vi "Configure Channels.vi"(8 "error in":errorcluster, 11 "AI DAQmx CFG in":refnum<class "AI DAQmx Cont CFG.lvclass">) -> (0 "error out":errorcluster, 3 "AI DAQmx CFG out":refnum<class "AI DAQmx Cont CFG.lvclass">)   [LabVIEW 2023, in "AI DAQmx Cont CFG.lvclass"]
uses:
  AI DAQmx Cont CFG.lvclass
  D:/git/HAL/HAL GOOP4/Configuration/Configuration JSON/Configuration JSON Base/CFG JSON.lvclass
  D:/git/HAL/HAL GOOP4/DAQmx/DAQmx Base CFG/DAQmx Base CFG.lvclass
  DAQmx/DAQmx Base CFG/DAQmx Base CFG.lvclass/DAQmx Base CFG.ctl
  Configuration/Configuration JSON/Configuration JSON Base/CFG JSON.lvclass/CFG JSON.ctl
  AI DAQmx Cont CFG.lvclass/AI DAQmx Cont CFG.ctl
  400a6ce3-2820-48d5-b38a-88c74ea68e48.vi
  <vilib>/JDP Science/JSONtext/Find Item.vi
  <vilib>/JDP Science/JSONtext/Next JSON Value.vi
  <vilib>/JDP Science/JSONtext/String Subset.vi
  <vilib>/JDP Science/JSONtext/Parsing/Advance past next JSON Value (inlined COPY).vi
  <vilib>/JDP Science/JSONtext/Parsing/Advance past whitespace.vi
  <vilib>/JDP Science/JSONtext/Parsing/Advance past String.vi
  <vilib>/JDP Science/JSONtext/Parsing/Advance past Number.vi
  <vilib>/JDP Science/JSONtext/Parsing/Advance past Line Ending.vi
  <vilib>/JDP Science/JSONtext/Parsing/Parse Full Path or Item Name.vi
  <vilib>/JDP Science/JSONtext/Parsing/Advance past Array.vi
  <vilib>/JDP Science/JSONtext/Parsing/Advance past Object.vi
  <vilib>/JDP Science/JSONtext/support/Error Cluster From Code.vi
  <vilib>/JDP Science/JSONtext/Offset/Find Item Locations by Path.vi
  <vilib>/JDP Science/JSONtext/JSON text to Variant.vi
  <vilib>/Utility/error.llb/Error Cluster From Error Code.vi
  <vilib>/DAQmx/create/channels.llb/DAQmx Create Channel (AI-Current-Basic).vi
  <vilib>/JDP Science/JSONtext/LVClass Serializer/JSONtext LVClass Serializer.lvclass
  <vilib>/ErrorRing/Error Ring.xnode
  DAQmx/BufferLastReadingsDBL/BufferLastReadsDBL.lvclass
  Configuration/Configuration JSON/Configuration JSON Base/CFG JSON.lvclass
  DAQmx/DAQmx Base CFG/DAQmx Base CFG.lvclass
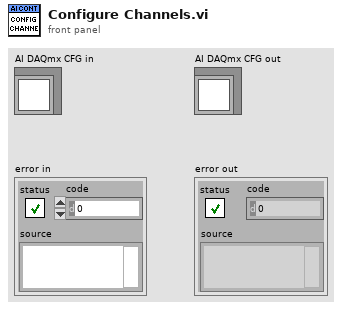
[diagram p1: front panel]
types:
  T1 = cluster{"Name":string, "Enabled":bool, "Max Value":dbl, "Min Value":dbl, "Input Terminal CFG":string, "Units":string, "Shunt Resistor Location":string, "External Shunt Resistor Value":dbl}[]
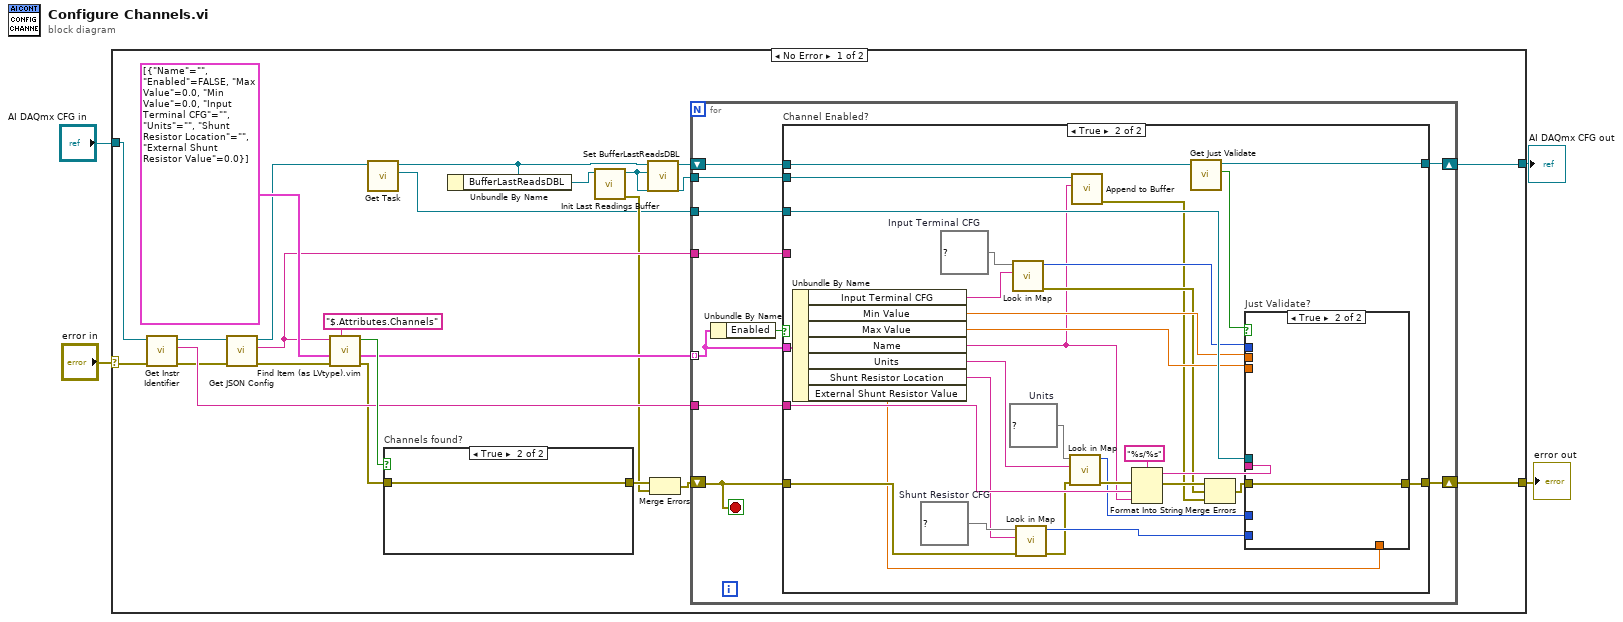
[diagram p0: block diagram]
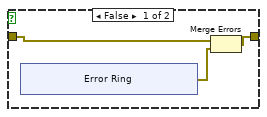
[diagram p2: hidden frame]
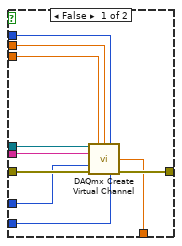
[diagram p4: hidden frame]
diagram:
  n1 = case shown="No Error" "error in" {
    selector: "error in" -> [w20 w89]
    tunnel: "AI DAQmx CFG in" -> [w17 w90]
    tunnel: [w21 w89] -> w2
    tunnel: [w16 w90] -> w1
    frame No Error {
      n2 = call-dynamic "Get Instr Identifier.vi"("error in (no error)"=w20, "Configuration Base in"=w17) -> ("error out"=w13:errorcluster, "Instr Ident"=w22:string, "Configuration Base out"=w23:refnum<class "AI DAQmx Cont CFG.lvclass">)  [unwired: 7 in]
      n3 = call "Get JSON Config.vi"("CFG Base in"=w23) -> ("<JSON>Config>"=w19:string, "CFG Base out"=w12:refnum<class "AI DAQmx Cont CFG.lvclass">)  [unwired: 9 in]
      n4 = call "Find Item (as LVtype).vim"("$Path or Item Name"="$.Attributes.Channels", "error in (no error)"=w13, "Data Type and Default Value"=T1 [{"Name"="", "Enabled"=FALSE, "Max Value"=0.0, "Min Value"=0.0, "Input Terminal CFG"="", "Units"="", "Shunt Resistor Location"="", "External Shunt Resistor Value"=0.0}], "JSON"=w19) -> ("error out"=w14:errorcluster, "Data"=w18:T1, "Found"=w25:bool)  [unwired: 4 in, 1 out]
      n5 = call "Get Task.vi"("DAQmx Base CFG in"=w12) -> ("Task"=w9:refnum<k21>, "DAQmx Base CFG out"=w6:refnum<class "AI DAQmx Cont CFG.lvclass">)  [unwired: 9 in]
      n6 = case "Channels found?" shown="True" w25 {
        tunnel: w14 -> [w29 w35]
        tunnel: [w27 w35] -> w15
        frame False {
          n7 = xnode "Error Ring"() -> ("error out"=w28:errorcluster)
          n8 = Merge Errors(w29, w28) -> (w27:errorcluster)
        }
        frame True {
        }
      }
      n9 = Unbundle By Name(w6) -> ("BufferLastReadsDBL"=w5:refnum<class "BufferLastReadsDBL.lvclass">)
      n10 = call-dynamic "Init Last Readings Buffer.vi"("BufferLastReadingsDBL in"=w5) -> ("error out"=w10:errorcluster, "BufferLastReadingsDBL out"=w7:refnum<class "BufferLastReadsDBL.lvclass">)  [unwired: 9 in]
      n11 = call "Set BufferLastReadsDBL.vi"("BufferLastReadings DBL"=w7, "AI DAQmx Cont CFG in"=w6) -> ("AI DAQmx Cont CFG out"=w8:refnum<class "AI DAQmx Cont CFG.lvclass">)  [unwired: 9 in]
      n12 = Merge Errors(w15, w10) -> (w11:errorcluster)
      n13 = for {
        tunnel: w18 -> [w42] mode=indexing
        shift-right: [w45] -> w21
        shift-left: w11 -> [w44]
        tunnel: w22 -> [w43]
        tunnel: w19 -> [w41]
        tunnel: w9 -> [w40]
        shift-right: [w39] -> w16
        shift-left: w8 -> [w38]
        tunnel: w7 -> [w36]
        stop <- w44 stop-if-true
        n14 = Unbundle By Name(w42) -> ("Enabled"=w37:bool)
        n15 = case "Channel Enabled?" shown="True" w37 {
          tunnel: [w47 w76] -> w45
          tunnel: w44 -> [w47 w54]
          tunnel: w43 -> [_ w70]
          tunnel: w42 -> [_ w77]
          tunnel: [w46 w73] -> w39
          tunnel: w41 -> [_ _]
          tunnel: w40 -> [_ w75]
          tunnel: w38 -> [w46 w74]
          tunnel: w36 -> [_ w50]
          frame False {
          }
          frame True {
            w58 = map{string, i32} {"External"=10167, "Internal"=10200, "default"=-1}  # Shunt Resistor CFG
            w64 = map{string, i32} {"Amps"=10342, "From Custom Scale"=10065}  # Units
            w66 = map{string, i32} {"Differential"=10106, "NRSE"=10078, "Pseudodifferential"=12529, "RSE"=10083, "default"=-1}  # Input Terminal CFG
            n16 = Unbundle By Name(w77) -> ("Input Terminal CFG"=w65:string, "Min Value"=w62:dbl, "Max Value"=w61:dbl, "Name"=w49:string, "Units"=w59:string, "Shunt Resistor Location"=w51:string, "External Shunt Resistor Value"=w52:dbl)
            n17 = call "Look in Map.vi"("Key"=w65, "Map"=w66) -> ("error out"=w57:errorcluster, "Value"=w63:i32)  [unwired: 8 in]
            n18 = call "Look in Map.vi"("error in"=w54, "Key"=w51, "Map"=w58) -> ("error out"=w53:errorcluster, "Value"=w55:i32)  [unwired: 7 in]
            n19 = call "Look in Map.vi"("error in"=w53, "Key"=w59, "Map"=w64) -> ("error out"=w60:errorcluster, "Value"=w56:i32)  [unwired: 7 in]
            n20 = call-dynamic "Append to Buffer.vi"("Channel"=w49, "BufferLastReadingsDBL in"=w50) -> ("error out"=w48:errorcluster)  [unwired: 8 in, 1 out]
            n21 = Format Into String(format string="%s/%s", error in=w60, w70, w49) -> (resulting string=w68:string, error out=w69:errorcluster)  [unwired: 1 in]
            n22 = call "Get Just Validate.vi"("CFG JSON Base in"=w74) -> ("Just Validate"=w72:bool, "CFG JSON Base out"=w73:refnum<class "AI DAQmx Cont CFG.lvclass">)  [unwired: 9 in]
            n23 = Merge Errors(w69, w57, w48) -> (w67:errorcluster)
            n24 = case "Just Validate?" shown="True" w72 {
              tunnel: w67 -> [w87 w88]
              tunnel: w68 -> [w84 _]
              tunnel: w75 -> [w86 _]
              tunnel: [w85 w88] -> w76
              tunnel: w63 -> [w83 _]
              tunnel: w62 -> [w82 _]
              tunnel: w61 -> [w81 _]
              tunnel: w56 -> [w80 _]
              tunnel: w55 -> [w79 _]
              tunnel: w52 -> [w78 _]
              frame False {
                n25 = call-poly <vilib>:"DAQmx Create Virtual Channel.vi"("task in"=w86, "maximum value"=w81, "minimum value"=w82, "input terminal configuration"=w83, "physical channels"=w84, "external shunt resistor value"=w78, "units"=w80, "error in"=w87, "shunt resistor location"=w79) -> ("error out"=w85:errorcluster)  [unwired: 5 in, 1 out]
              }
              frame True {
              }
            }
          }
        }
      }
    }
    frame Error {
    }
  }
  "error out" <- w2
  "AI DAQmx CFG out" <- w1
